vi "Available Black Levels.vi"(8 "error in (no error)":errorcluster, 11 "Camera in":refnum<class "Camera.lvclass">) -> (0 "error out":errorcluster, 2 "Available Black Levels":string[](array[string]), 3 "Camera":refnum<class "Camera.lvclass">)   [LabVIEW 2020, in "Camera.lvclass"]
uses:
  Camera.lvclass
  Camera.lvclass/Camera.ctl
  bin/gindustrialcam_32-1.dll
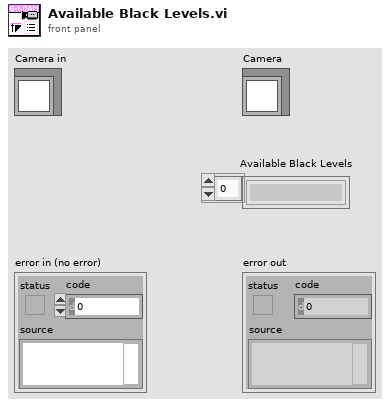
[diagram p1: front panel]
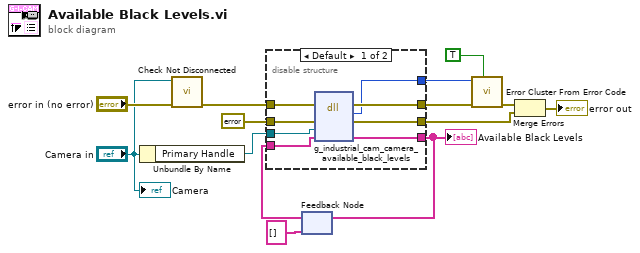
[diagram p0: block diagram]
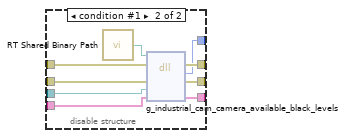
[diagram p2: hidden frame]
diagram:
  n1 = Unbundle By Name("Camera in") -> ("Primary Handle"=w3:refnum<data-value>)
  n2 = call "Check Not Disconnected.vi"("error in (no error)"="error in (no error)", "Camera in"="Camera in") -> ("error out"=w2:errorcluster)  [unwired: 9 in]
  n3 = feedback #1(string[] []) -> (w5:string[])
  n4 = disable-structure shown="Default" {
    disable-tunnel: [w22 w31] -> w12
    disable-tunnel: [w21 w30] -> w11
    disable-tunnel: [w20 w29] -> w9
    disable-tunnel: errorcluster {"status"=FALSE, "code"=0, "source"=""} ("error constant") -> [w19 w28]
    disable-tunnel: w5 -> [w18 w27]
    disable-tunnel: [w17 w26] -> w4
    disable-tunnel: w3 -> [w16 w25]
    disable-tunnel: w2 -> [w15 w24]
    frame condition #0 (active) {
      n5 = dll-call lib="C:/serenial/lib/g-industrial-camera/LabVIEW/g_industrial_cam/bin/gindustrialcam_*-1.*" fn="g_industrial_cam_camera_available_black_levels"(error in=w15, "err"=w19, "edvr"=w16, "formats"=w18) -> (error out=w22:errorcluster, "Mg_Error"=w21:i32, "err"=w20:errorcluster, "formats"=w17:string[])  [unwired: 3 in, 1 out]
    }
    frame condition #1 {
      n6 = call "RT Shared Binary Path.vi"() -> ("Path"=w23:path)
      n7 = dll-call lib="C:/serenial/lib/g-industrial-camera/LabVIEW/g_industrial_cam/bin/gindustrialcam_*-1.*" fn="g_industrial_cam_camera_available_black_levels"(path in=w23, error in=w24, "err"=w28, "edvr"=w25, "formats"=w27) -> (error out=w31:errorcluster, "Mg_Error"=w30:i32, "err"=w29:errorcluster, "formats"=w26:string[])  [unwired: 2 in, 1 out]
    }
  }
  "Available Black Levels" <- w4
  n8 = feedback-in #1(w4) -> ()
  n9 = call <vilib>:"Error Cluster From Error Code.vi"("show call chain? (False)"=TRUE, "error in (no error)"=w12, "error code (0)"=w11) -> ("error out"=w10:errorcluster)  [unwired: 6 in]
  n10 = Merge Errors(w10, w9) -> (→"error out":errorcluster)
  "Camera" <- "Camera in"
